vi "SquareBattle Main.vi"() -> ()   [LabVIEW 2015]
uses:
  Type Defs/Dashboard.ctl
  Type Defs/UI Refs.ctl
  SubVIs/Globals.vi
  Type Defs/SB Type Defs.lvlib
  SubVIs/SB SubVIs.lvlib
  Endigit Library/Endigit.lvlib
panel:
  out "Elapsed Time":u32
  in  "Dashboard":T1[](array[typedef]) {"Player" items=["<Select a Square>", "Assassin", "Cautious Wolf", "Crosswinds", "Demo", "Expand", "Formation", "Galaxy", "Impenetrable", "Pattern 1", "Pattern 2", "Pattern 3", "Pattern 4", "Pattern 5", "Pic", "Pinwheel", "Rain", "SVoT", "Sentinel", "Sir Robin"]}
  out "Actual Speed":dbl format="%.1f"
  out "Round":i32
  in  "Board size":i32=150
  in  "End Battle":bool
  in  "Game Speed":u32(slide)=1000 caption="Game Speed (rounds/second)" min=1 max=1000 step=1 scale=1.0..1000.0
  in  "Start Battle":bool
  out "Battlefield":i32[][](graph)
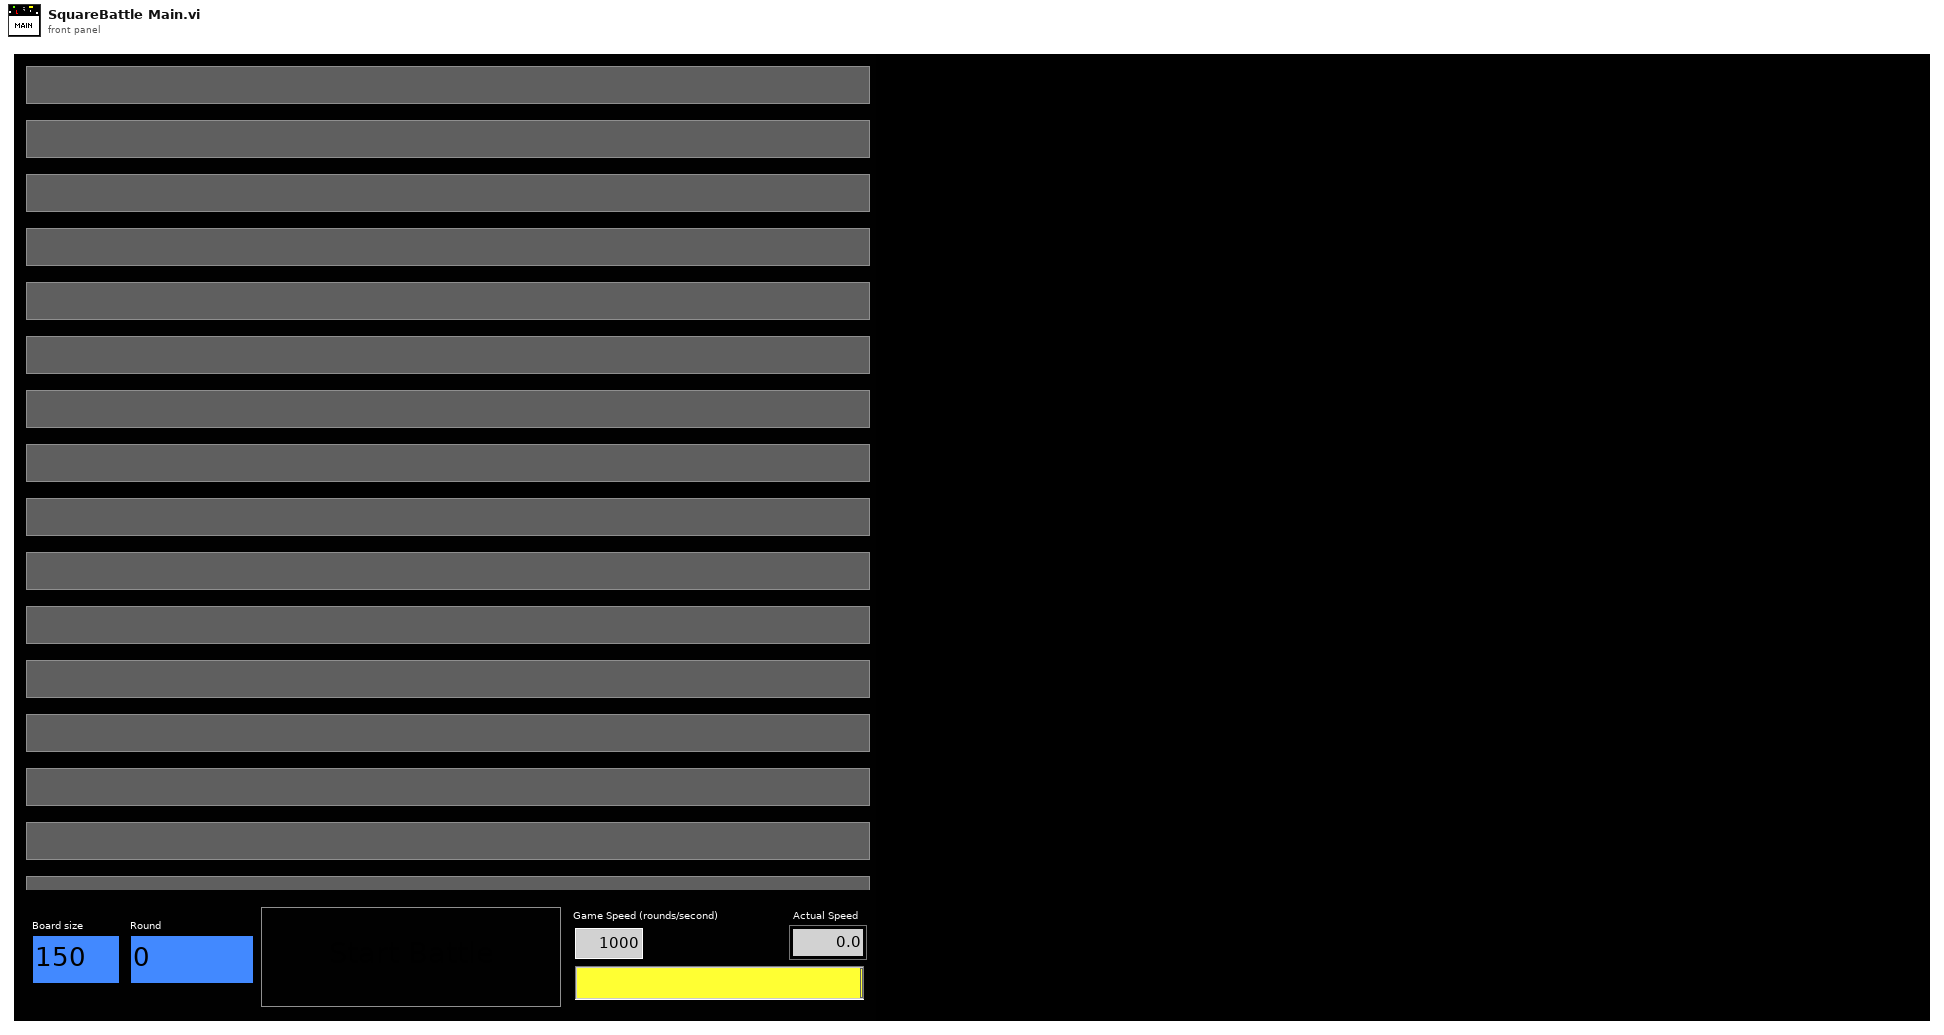
[diagram p1: front panel]
types:
  T1 = typedef "SB Type Defs.lvlib/Dashboard.ctl" = cluster{"Color":u32, "Player":i32, "Status":string, "Stats":string}
  T2 = typedef "SB Type Defs.lvlib/UI Refs.ctl" = cluster{"Battlefield":refnum<vi>, "Dashboard":refnum<vi>, "End Battle":refnum<vi>}
  T3 = typedef "LVPoint32TypeDef.ctl" = cluster{"Horizontal":i32, "Vertical":i32}
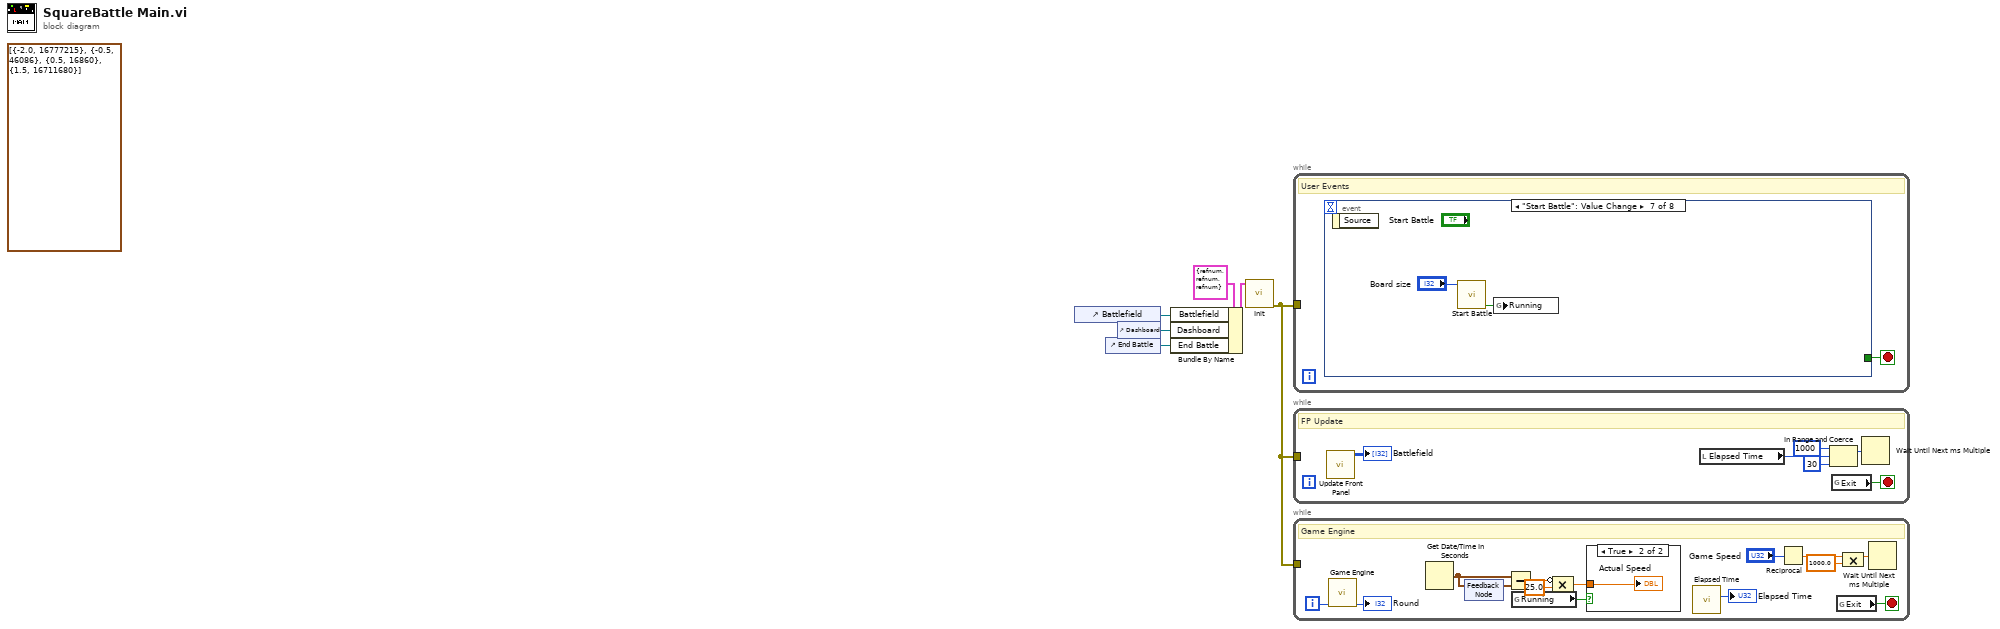
[diagram p0: block diagram]
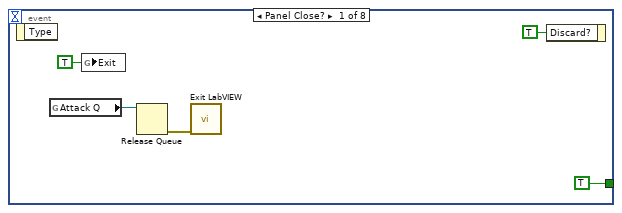
[diagram p3: hidden frame]
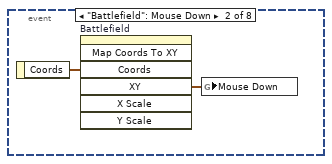
[diagram p4: hidden frame]
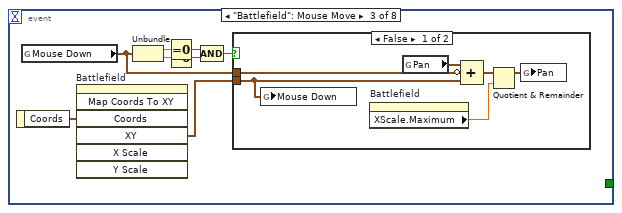
[diagram p5: hidden frame]
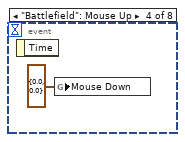
[diagram p7: hidden frame]
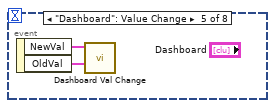
[diagram p8: hidden frame]
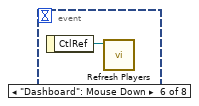
[diagram p9: hidden frame]
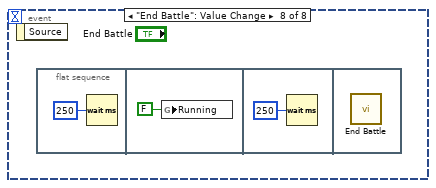
[diagram p10: hidden frame]
diagram:
  (unwired) cluster{dbl, u32}[] [{-2.0, 16777215}, {-0.5, 46086}, {0.5, 16860}, {1.5, 16711680}] ("Z Scale.Marker Values[]")
  n1 = control-ref of="Battlefield"() -> (w3:refnum<vi>)
  n2 = control-ref of="End Battle"() -> (w6:refnum<vi>)
  n3 = control-ref of="Dashboard"() -> (w4:refnum<vi>)
  n4 = Bundle By Name(cluster=T2 {"Battlefield"=refnum, "Dashboard"=refnum, "End Battle"=refnum} ("UI Refs"), "Battlefield"=w3, "Dashboard"=w4, "End Battle"=w6) -> (w2:T2)
  n5 = call "Init.vi"("UI Refs"=w2) -> ("Error Out"=w1:errorcluster)  [unwired: 10 in]
  n6 = while {
    tunnel: w1 -> [_]
    stop <- w7 stop-if-true
    # "User Events"
    n7 = event shown="[6] \"Start Battle\": Value Change" {
      selector: _ -> [_ _ _ _ _ _ _ _]
      dyn-events: _ -> [_ _ _ _ _ _ _ _]
      timeout: _ -> [_ _ _ _ _ _ _ _]
      tunnel: [TRUE _ _ _ _ _ _ _] -> w7
      event Panel Close? {
        n8 = event-data() -> ()  [unwired: 1 in, 1 out]
        n9 = global read "Globals.vi" "Attack Q"() -> (w10:refnum<queue>)
        n10 = global write "Globals.vi" "Exit"(TRUE ("Exit")) -> ()
        n11 = Release Queue(queue=w10) -> (error out=w8:errorcluster)  [unwired: 2 in, 2 out]
        n12 = call "Exit LabVIEW.vi"("Error (Dependency Only)"=w8) -> ()  [unwired: 11 in]
        n13 = event-data("Discard?"=TRUE) -> ()  [unwired: 1 in, 1 out]
      }
      event "Battlefield": Mouse Down {
        n14 = event-data() -> ("Coords"=w14:T3)  [unwired: 1 in]
        n15 = invoke on="Battlefield" class="IntGraph (strict)" method="Map Coords To XY"("Coords"=w14) -> ("XY"=w13:cluster{"X":dbl, "Y":dbl})  [unwired: 6 in, 6 out]
        n16 = global write "Globals.vi" "Mouse Down"(w13) -> ()
      }
      event "Battlefield": Mouse Move {
        n17 = event-data() -> ("Coords"=w17:T3)  [unwired: 1 in]
        n18 = global read "Globals.vi" "Mouse Down"() -> (w15:cluster{"X":dbl, "Y":dbl})
        n19 = invoke on="Battlefield" class="IntGraph (strict)" method="Map Coords To XY"("Coords"=w17) -> ("XY"=w16:cluster{"X":dbl, "Y":dbl})  [unwired: 6 in, 6 out]
        n20 = Unbundle(w15) -> ("X"=w22:dbl, "Y"=w21:dbl)
        n21 = Equal To 0?(x=w22) -> (x = 0?=w20:bool)
        n22 = Equal To 0?(x=w21) -> (x = 0?=w19:bool)
        n23 = Compound Arithmetic op=AND(w20, w19) -> (w18:bool)
        n24 = case shown="False" w18 {
          tunnel: w16 -> [w23 _]
          tunnel: w15 -> [w27 _]
          frame False {
            n25 = global write "Globals.vi" "Mouse Down"(w23) -> ()
            n26 = property on="Battlefield" class="IntGraph (strict)"() -> ("XScale.Maximum"=w28:dbl)  [unwired: 2 in, 2 out]
            n27 = global read "Globals.vi" "Pan"() -> (w25:cluster{"Horizontal":dbl, "Vertical":dbl})
            n28 = Compound Arithmetic op=ADD(w25, invert w27, w23) -> (w26:cluster{dbl, dbl})
            n29 = Quotient & Remainder(x=w26, y=w28) -> (x-y*floor(x/y)=w24:cluster{dbl, dbl})  [unwired: 1 out]
            n30 = global write "Globals.vi" "Pan"(w24) -> ()
          }
          frame True {
          }
        }
      }
      event "Battlefield": Mouse Up {
        n31 = event-data() -> ()  [unwired: 1 in, 1 out]
        n32 = global write "Globals.vi" "Mouse Down"(cluster{"X":dbl, "Y":dbl} {"X"=0.0, "Y"=0.0} ("Mouse Down")) -> ()
      }
      event "Dashboard": Value Change {
        n33 = event-data() -> ("NewVal"=w30:T1[], "OldVal"=w31:T1[])  [unwired: 1 in]
        n34 = call "Dashboard Val Change.vi"("OldVal"=w31, "NewVal"=w30) -> ()  [unwired: 10 in]
      }
      event "Dashboard": Mouse Down {
        n35 = event-data() -> ("CtlRef"=w32:refnum<vi>)  [unwired: 1 in]
        n36 = call "Refresh Players.vi"("Dashboard"=w32) -> ()  [unwired: 10 in, 1 out]
      }
      event "Start Battle": Value Change {
        n37 = event-data() -> ()  [unwired: 1 in, 1 out]
        n38 = call "Start Battle.vi"("Board Size"="Board size") -> ("Start"=w33:bool)  [unwired: 10 in]
        n39 = global write "Globals.vi" "Running"(w33) -> ()
      }
      event "End Battle": Value Change {
        n40 = event-data() -> ()  [unwired: 1 in, 1 out]
        n41 = flat-sequence {
          frame #0 {
            n42 = Wait (ms)(milliseconds to wait=u32 250) -> ()  [unwired: 1 out]
          }
          frame #1 {
            n43 = global write "Globals.vi" "Running"(FALSE ("Running")) -> ()
          }
          frame #2 {
            n44 = Wait (ms)(milliseconds to wait=u32 250) -> ()  [unwired: 1 out]
          }
          frame #3 {
            n45 = call "End Battle.vi"() -> ()  [unwired: 12 in]
          }
        }
      }
    }
  }
  n46 = while {
    tunnel: w1 -> [_]
    stop <- w39 stop-if-true
    # "FP Update"
    n47 = call "Update Front Panel.vi"() -> ("Battlefield"=→"Battlefield":i32[][])  [unwired: 11 in]
    n48 = local read "Elapsed Time"() -> (w40:u32)
    n49 = In Range and Coerce(upper limit=u32 1000 ("millisecond multiple"), x=w40, lower limit=u32 30) -> (coerced(x)=w43:u32)  [unwired: 1 out]
    n50 = global read "Globals.vi" "Exit"() -> (w39:bool)
    n51 = Wait Until Next ms Multiple(millisecond multiple=w43) -> ()  [unwired: 1 out]
  }
  n52 = while {
    tunnel: w1 -> [_]
    i -> [w55]
    stop <- w57 stop-if-true
    # "Game Engine"
    n53 = call "Game Engine.vi"("Iteration"=w55) -> ("Round"=→"Round":i32)  [unwired: 10 in]
    n54 = Get Date/Time In Seconds() -> (seconds since 1Jan1904=w49:timestamp)
    n55 = feedback-in #1(w49) -> ()
    n56 = feedback #1() -> (w48:timestamp)  [unwired: 1 in]
    n57 = Subtract(x=w49, y=w48) -> (x-y=w47:dbl)
    n58 = global read "Globals.vi" "Running"() -> (w50:bool)
    n59 = Compound Arithmetic op=MULTIPLY(invert w47, 25.0 ("value")) -> (w45:dbl)
    n60 = case shown="True" w50 {
      tunnel: w45 -> [_ w58]
      frame False {
      }
      frame True {
        "Actual Speed" <- w58
      }
    }
    n61 = call "Elapsed Time.vi"() -> ("Elapsed Time"=→"Elapsed Time":u32)  [unwired: 11 in]
    n62 = Reciprocal(x="Game Speed") -> (1/x=w54:dbl)
    n63 = global read "Globals.vi" "Exit"() -> (w57:bool)
    n64 = Compound Arithmetic op=MULTIPLY(w54, 1000.0 ("value")) -> (w53:dbl)
    n65 = Wait Until Next ms Multiple(millisecond multiple=w53) -> ()  [unwired: 1 out]
  }
